vi "Read cluster.vi"(11 "ValveModbus in":refnum<class "ValveModbus.lvclass">) -> (2 "cluster":T1, 3 "ValveModbus out":refnum<class "ValveModbus.lvclass">)   [LabVIEW 2019, in "ValveModbus.lvclass"]
uses:
  ValveModbus.lvclass
  modbus engine custom/MB_ENGINE_class/Settings.ctl
  ValveModbus.lvclass/ValveModbus.ctl
  modbus engine custom/MB_ENGINE_class/MB_ENGINE.lvclass
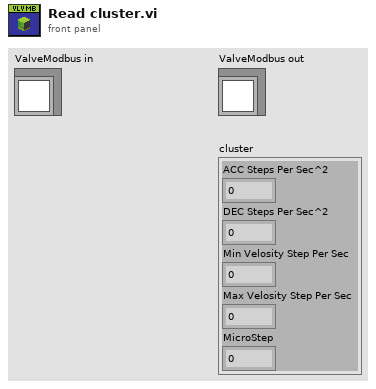
[diagram p1: front panel]
types:
  T1 = typedef "MB_ENGINE.lvclass/Settings.ctl" = cluster{"ACC Steps Per Sec^2":u16, "DEC Steps Per Sec^2":u16, "Min Velosity Step Per Sec":u16, "Max Velosity Step Per Sec":u16, "MicroStep":u16}
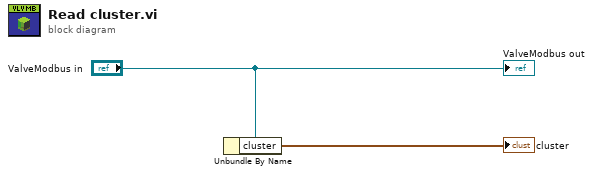
[diagram p0: block diagram]
diagram:
  n1 = Unbundle By Name("ValveModbus in") -> ("cluster"=→"cluster":T1)
  "ValveModbus out" <- "ValveModbus in"
